vi "Logging Utility.vi"(0 "Username":string, 1 "Z Coord":dbl, 2 "Y Coord":dbl, 3 "X Coord":dbl, 4 "Temperature":dbl, 5 "Event":string, 6 "Timestamp":timestamp, 7 "Path":path) -> ()   [LabVIEW 2017]
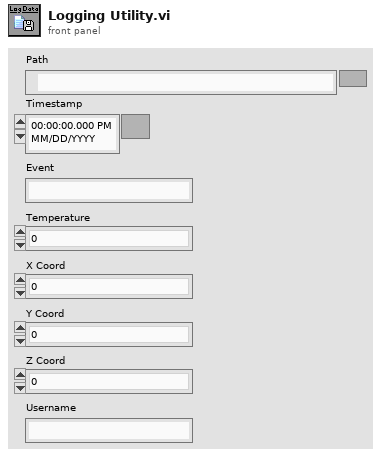
[diagram p1: front panel]
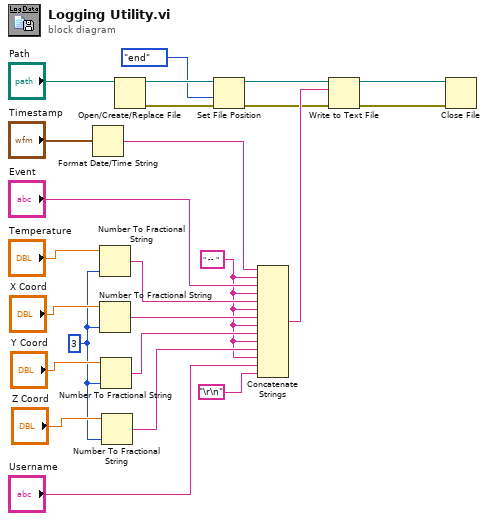
[diagram p0: block diagram]
diagram:
  w1 = " -- "
  w2 = 3
  n1 = Format Date/Time String(seconds (now)="Timestamp") -> (date/time string=w11:string)  [unwired: 2 in]
  n2 = Number To Fractional String(number="Temperature", precision (6)=w2) -> (F-format string=w9:string)  [unwired: 2 in]
  n3 = Number To Fractional String(number="X Coord", precision (6)=w2) -> (F-format string=w8:string)  [unwired: 2 in]
  n4 = Number To Fractional String(number="Y Coord", precision (6)=w2) -> (F-format string=w7:string)  [unwired: 2 in]
  n5 = Number To Fractional String(number="Z Coord", precision (6)=w2) -> (F-format string=w6:string)  [unwired: 2 in]
  n6 = Open/Create/Replace File(file path (use dialog)="Path") -> (refnum out=w17:refnum<file>, error out=w15:errorcluster)  [unwired: 5 in, 1 out]
  n7 = Set File Position(refnum=w17, from (0:start)=enum16{"start", "end", "current"}."end", error in=w15) -> (refnum out=w16:refnum<file>, error out=w14:errorcluster)  [unwired: 1 in]
  n8 = Concatenate Strings(w11, w1, "Event", w1, w9, w1, w8, w1, w7, w1, w6, w1, "Username", "\r\n") -> (w19:string)
  n9 = Write to Text File(file (use dialog)=w16, text=w19, error in=w14) -> (refnum out=w22:refnum<file>, error out=w23:errorcluster)  [unwired: 1 in, 1 out]
  n10 = Close File(refnum=w22, error in=w23) -> ()  [unwired: 2 out]
